vi "comms_BT_Send_Com.vi"(8 "error in":errorcluster, 9 "Buffer Clear?":bool, 10 "Command":string, 11 "connection ID":refnum<k31>) -> (0 "error out":errorcluster, 2 "Response":string, 3 "connection ID out":refnum<k31>)   [LabVIEW 2016]
panel:
  out "Cleared Data":string
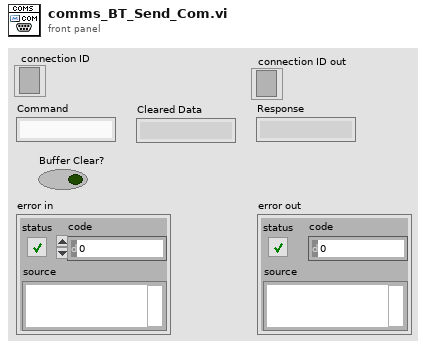
[diagram p1: front panel]
types:
  T1 = enum16{"Standard", "Buffered", "CRLF", "Immediate"}
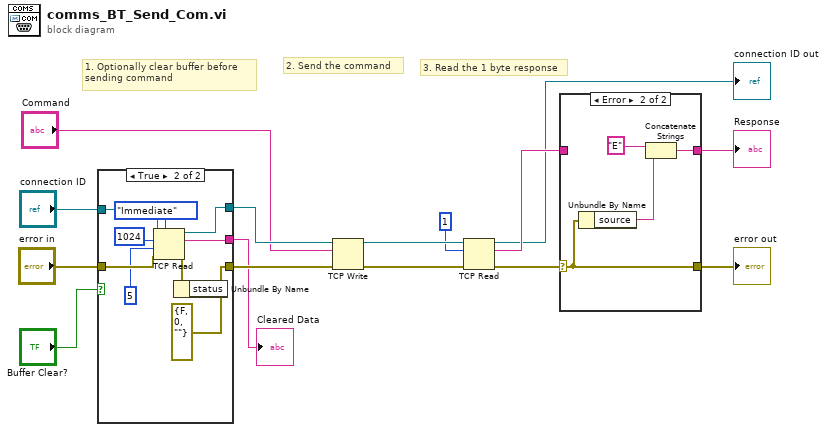
[diagram p0: block diagram]
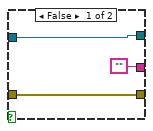
[diagram p3: hidden frame]
diagram:
  # "3. Read the 1 byte response"
  # "2. Send the command"
  # "1. Optionally clear buffer before \nsending command"
  n1 = case shown="True" "Buffer Clear?" {
    tunnel: [w17 w25] -> w10
    tunnel: "error in" -> [w18 w27]
    tunnel: [w18 errorcluster {"status"=FALSE, "code"=0, "source"=""} ("error in")] -> w9
    tunnel: "connection ID" -> [w17 w26]
    tunnel: ["" w19] -> w1
    frame False {
    }
    frame True {
      n2 = TCP Read(connection ID=w26, bytes to read=1024, error in (no error)=w27, 7:T1."Immediate" ("mode (standard)"), 9:5 ("timeout ms (25000)")) -> (connection ID out=w25:refnum<k31>, data out=w19:string, error out=w22:errorcluster)
      n3 = Unbundle By Name(w22) -> ()  [unwired: 1 out]
    }
  }
  "Cleared Data" <- w1
  n4 = TCP Write(connection ID=w10, data in="Command", error in (no error)=w9) -> (connection ID out=w6:refnum<k31>, error out=w7:errorcluster)  [unwired: 1 in, 1 out]
  n5 = TCP Read(connection ID=w6, bytes to read=u32 1 ("byte count"), error in (no error)=w7) -> (connection ID out=→"connection ID out":refnum<k31>, data out=w5:string, error out=w2:errorcluster)  [unwired: 2 in]
  n6 = case shown="Error" w2 {
    selector: w2 -> [w29 w33]
    tunnel: [w29 w33] -> w13
    tunnel: w5 -> [w28 _]
    tunnel: [w28 w32] -> w12
    frame No Error {
    }
    frame Error {
      n7 = Unbundle By Name(w33) -> ("source"=w31:string)
      n8 = Concatenate Strings("E", w31) -> (w32:string)
    }
  }
  "error out" <- w13
  "Response" <- w12
